vi "Get Command Documentation.vi"(0 "SLSC Remote in":refnum<class "SLSC Remote.lvclass">, 5 "command":refnum<k21>, 11 "error in (no error)":errorcluster) -> (4 "SLSC Remote out":refnum<class "SLSC Remote.lvclass">, 6 "command out":refnum<k21>, 10 "Cmd.Doc":string, 15 "error out":errorcluster)   [LabVIEW 2015, in "SLSC Remote.lvclass"]
uses:
  SLSC Remote.lvclass
  <vilib>/NI/i3 JSON/JSON Generation/Create Value Files/Create Value - Object.vi
  <vilib>/NI/i3 JSON/JSON Generation/Add Object Parameter Files/Add Object Parameter - String.vi
  <vilib>/NI/NI JSONRPC Server Framework/Classes/Server/Format Client Request (Auto-Increment).vi
  <vilib>/httpClient/POSTBuffer.vi
  <vilib>/NI/i3 JSON/JSON Parsing/Get Object Parameter Files/Get Object Parameter - String.vi
  <vilib>/NI/NI JSONRPC Server Framework/Classes/Server/JSONRPC Server.lvclass
  <vilib>/NI/i3 JSON/i3-json.lvlib
  <vilib>/httpClient/LabVIEWHTTPClient.lvlib
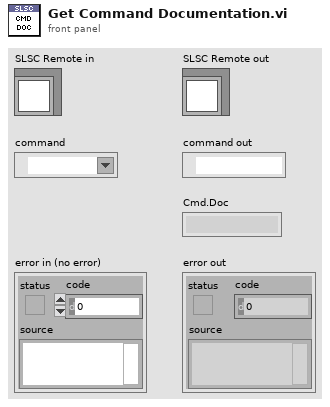
[diagram p1: front panel]
types:
  T1 = typedef "LabVIEWHTTPClient.lvlib/ClientHandle.ctl" = refnum<k1>
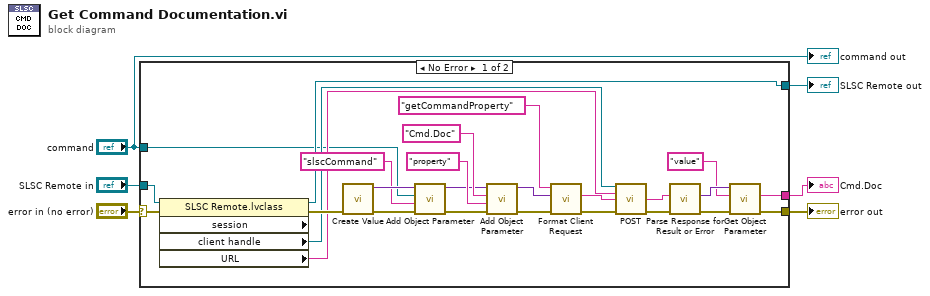
[diagram p0: block diagram]
diagram:
  n1 = case shown="No Error" "error in (no error)" {
    selector: "error in (no error)" -> [w29 w33]
    tunnel: "SLSC Remote in" -> [w31 w34]
    tunnel: [w30 w34] -> w3
    tunnel: [w17 w33] -> w1
    tunnel: [w16 _] -> w2
    tunnel: "command" -> [w10 _]
    frame No Error {
      n2 = property class="SLSC Remote.lvclass" props=["session", "client handle", "URL"](reference=w31, error in=w29) -> (reference out=w30:refnum<class "SLSC Remote.lvclass">, error out=w28:errorcluster, "client handle"=w24:T1, "URL"=w23:string)  [unwired: 1 out]
      n3 = call-poly <vilib>:"Create Value.vi"("error in (no error)"=w28) -> ("error out"=w27:errorcluster, "JSON Tree"=w32:variant)  [unwired: 9 in]
      n4 = call-poly <vilib>:"Add Object Parameter.vi"("error in (no error)"=w27, "Name"="slscCommand", "String"=w10, "JSON Tree in (JSON Object)"=w32) -> ("error out"=w7:errorcluster, "JSON Tree out (JSON Object)"=w8:variant)  [unwired: 6 in]
      n5 = call-poly <vilib>:"Add Object Parameter.vi"("error in (no error)"=w7, "Name"="property", "String"="Cmd.Doc", "JSON Tree in (JSON Object)"=w8) -> ("error out"=w13:errorcluster, "JSON Tree out (JSON Object)"=w14:variant)  [unwired: 6 in]
      n6 = call-poly <vilib>:"Format Client Request.vi"("error in (no error)"=w13, "params"=w14, "method"="getCommandProperty") -> ("error out"=w22:errorcluster, "Request String"=w25:string)  [unwired: 7 in]
      n7 = call-poly <vilib>:"POST.vi"("client handle"=w24, "url"=w23, "buffer"=w25, "error in (no error)"=w22) -> ("body"=w21:string, "error out"=w20:errorcluster)  [unwired: 8 in, 2 out]
      n8 = call <vilib>:"Parse Response for Result or Error.vi"("error in"=w20, "Response String In"=w21) -> ("error out"=w18:errorcluster, "Result or Error Data"=w19:variant)  [unwired: 8 in]
      n9 = call-poly <vilib>:"Get Object Parameter.vi"("error in (no error)"=w18, "Parameter Name"="value", "JSON Tree In (JSON Object)"=w19) -> ("error out"=w17:errorcluster, "String Value"=w16:string)  [unwired: 5 in, 2 out]
    }
    frame Error {
    }
  }
  "error out" <- w1
  "SLSC Remote out" <- w3
  "Cmd.Doc" <- w2
  "command out" <- "command"
